vi "消息入队列函数.vi"(6 "优先入队列？":bool, 8 "错误输入（无错误）":errorcluster, 9 "消息数据":variant, 10 "message":string, 11 "队列输入":refnum<queue>) -> (0 "错误输出":errorcluster caption="error out", 3 "队列输出":refnum<queue>)   [LabVIEW 2013]
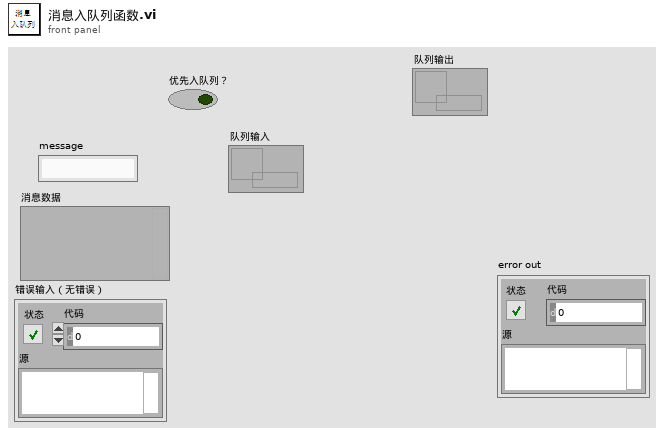
[diagram p1: front panel]
types:
  T1 = typedef "消息命令控件.ctl" = cluster{"message":string, "变体数据":variant}
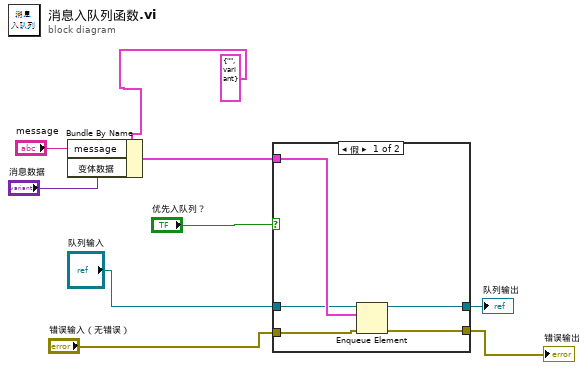
[diagram p0: block diagram]
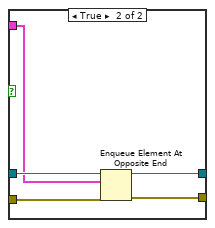
[diagram p2: hidden frame]
diagram:
  n1 = Bundle By Name(cluster=T1 {"message"="", "变体数据"=variant} ("命令消息"), "message"="message", "变体数据"="消息数据") -> (w8:T1)
  n2 = case shown="假" "优先入队列？" {
    tunnel: w8 -> [w14 w15]
    tunnel: "队列输入" -> [w13 w19]
    tunnel: [w12 w18] -> w1
    tunnel: "错误输入（无错误）" -> [w11 w17]
    tunnel: [w10 w16] -> w4
    frame False {
      n3 = Enqueue Element(queue=w13, element=w14, error in (no error)=w11) -> (queue out=w12:refnum<queue>, error out=w10:errorcluster)  [unwired: 1 in, 1 out]
    }
    frame True {
      n4 = Enqueue Element At Opposite End(queue=w19, element=w15, error in (no error)=w17) -> (queue out=w18:refnum<queue>, error out=w16:errorcluster)  [unwired: 1 in, 1 out]
    }
  }
  "错误输出" <- w4
  "队列输出" <- w1
